vi "BracePLUS_UI_Analysis.vi"(8 "error in":errorcluster, 11 "Path":path) -> (0 "error out":errorcluster)   [LabVIEW 2018]
uses:
  <vilib>/Math Plots/3D Math Plots/3D Surface/3D Surface XCtrl/3D Surface.xctl
  subVIs/calibration/FGVs/FGV States.ctl
  <vilib>/Utility/file.llb/Read Delimited Spreadsheet (I64).vi
  <vilib>/Math Plots/3D Math Plots/3D Surface/3D Surface Datatype/Public/Plot Helper (Matrix).vi
  <vilib>/Math Plots/3D Math Plots/3D Surface/3D Surface Datatype/3D Surface Datatype.lvclass
panel:
  in  "Quit":bool
  out "Time Frame":i32(slide) scale=0.0..975.0
  in  "Tab Control":T1(tab)
  out "3D Surface":refnum<class "3D Plot Datatype.lvclass">[](xcontrol)
  out "Z Time_Integral":refnum<class "3D Plot Datatype.lvclass">[](xcontrol)
  out "Data Packet":string
  out "Time":u32=4294745741
  out "Lookup Indices":i32[](array[numeric])=[0, 4, 8, 12, 1, 5, 9, 13, 16, 20, 24, 28, 17, 21, 25, 29, 15, 11, 7, 3, 14, 10, 6, 2, 31, 27, 23, 19, 30, 26, 22, 18, 32, 36, 40, 44, 33, 37, 41, 45, 48, 52, 56, 60, 49, 53, 57, 61, 47, 43, 39, 35, 46, 42, 38, 34, 63, 59, 55, 51, 62, 58, 54, 50, 64, 68, 72, 76, 65, 69, 73, 77, 80, 84, 88, 92, 81, 85, 89, 93, 79, 75, 71, 67, 78, 74, 70, 66, 95, 91, 87, 83, 94, 90, 86, 82, 96, 100, 104, 108, 97, 101, 105, 109, 112, 116, 120, 124, 113, 117, 121, 125, 111, 107, 103, 99, 110, 106, 102, 98, 127, 123, 119, 115, 126, 122, 118, 114]
  out "EOF?":bool
  in  "Start Z_Threshold":dbl=0.1 format="%#_13g"
  in  "Calibration File":string="Magboard_Btod_new_calib"
  in  "Gains":dbl[](array[numeric])=[0.751, 0.751, 1.21]
  in  "Upper Limit":dbl=5.0 format="%#_13g"
  in  "Lower Limit":dbl format="%#_13g"
  out "Filesize (bytes)":i64
  out "No. Packets":dbl
  out "Calibrated Output":dbl[][](array[numeric])
  out "B xyz":dbl[][](array[numeric]) format="%#.0f"
  # "ESCAPES: Analysis"
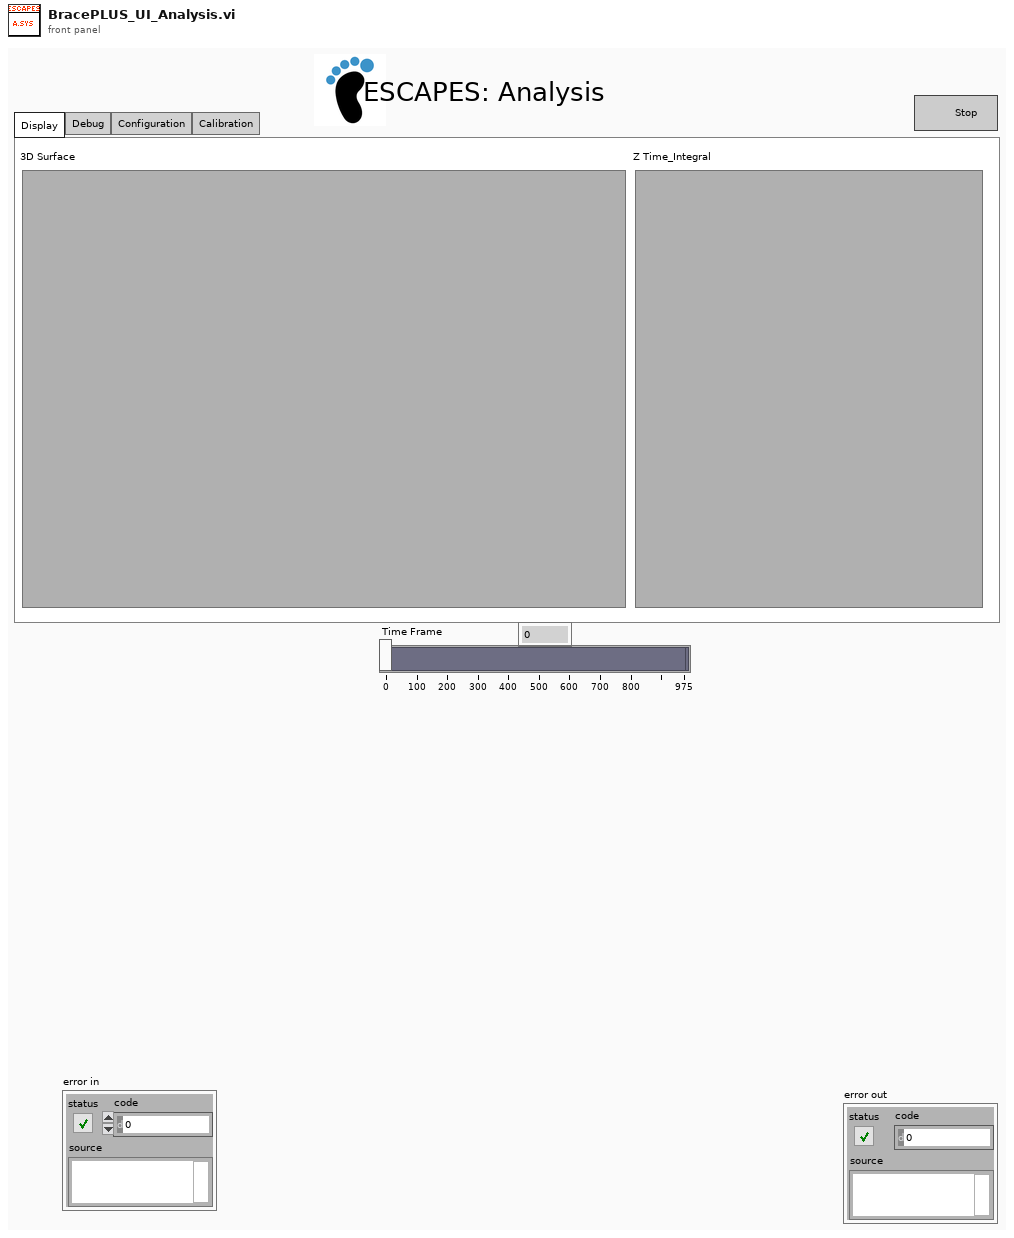
[diagram p1: front panel]
types:
  T1 = enum32{"Display", "Debug", "Configuration", "Calibration"}
  T2 = typedef "FGV States.ctl" = enum16{"Get", "Set", "Reset"}
  T3 = cluster{cluster{dbl[][], "Array":dbl[][]}, cluster{dbl[][], "Array":dbl[][]}, cluster{dbl[][], "Array":dbl[][]}, cluster{dbl[][], "Array":dbl[][]}}
  T4 = cluster{cluster{dbl[][], "Array":dbl[][]}, cluster{dbl[][], "Array":dbl[][]}, cluster{dbl[][], "Array":dbl[][]}, cluster{dbl[][], "Array":dbl[][]}}[]
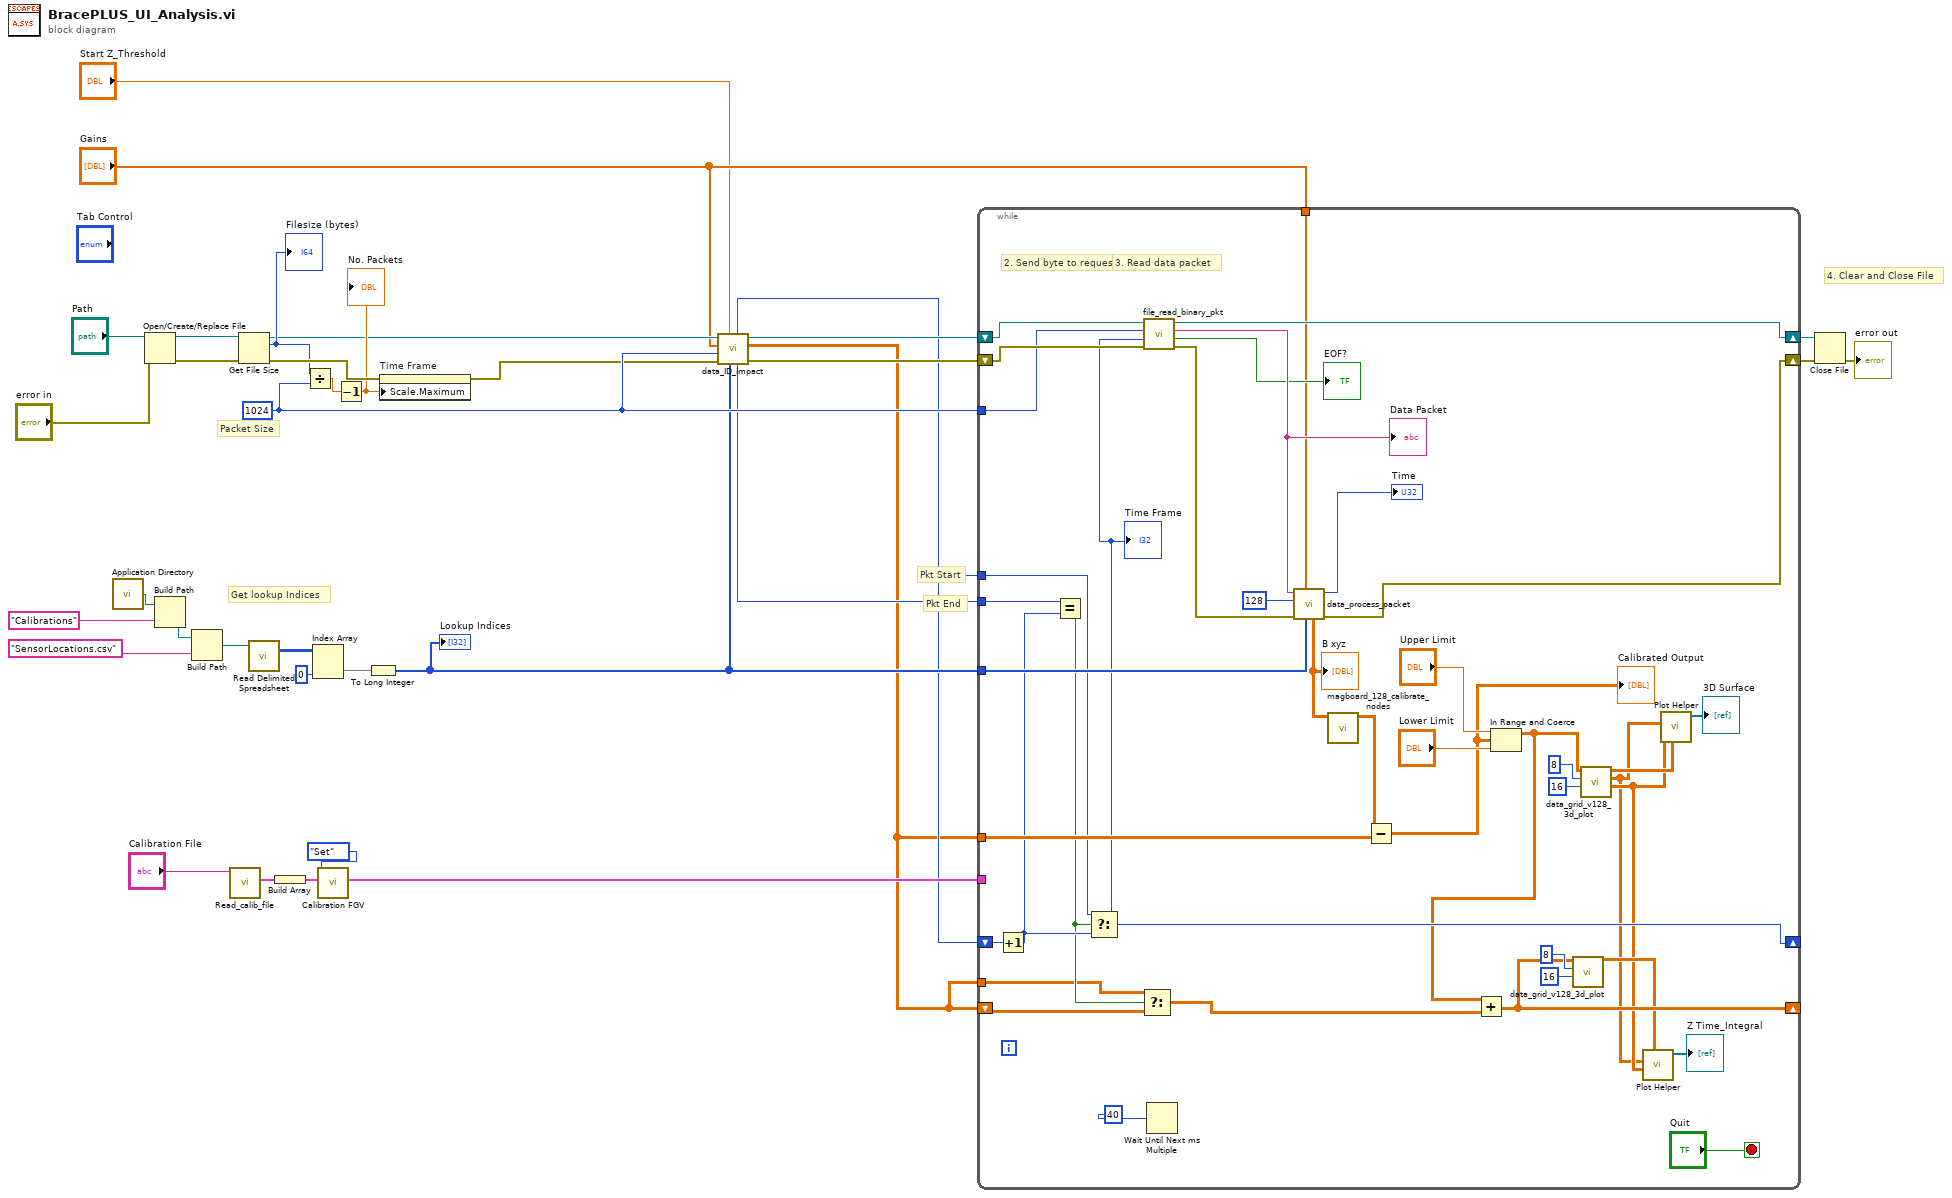
[diagram p0: block diagram]
diagram:
  w12 = 1024 ("count (1)")
  # "Pkt End"
  # "Pkt Start"
  # "Packet Size"
  # "Get lookup Indices"
  # "4. Clear and Close File"
  n1 = call <vilib>:"Application Directory.vi"() -> ("Application Directory"=w15:path)
  n2 = Open/Create/Replace File(file path (use dialog)="Path", error in="error in") -> (refnum out=w24:refnum<file>, error out=w23:errorcluster)  [unwired: 4 in, 1 out]
  n3 = Build Path(base path=w15, name or relative path="Calibrations" ("string")) -> (appended path=w17:path)
  n4 = Build Path(base path=w17, name or relative path="SensorLocations.csv" ("string")) -> (appended path=w14:path)
  n5 = call "Read_calib_file.vi"("string"="Calibration File") -> ("output cluster"=w32:T3)  [unwired: 6 in, 4 out]
  n6 = Get File Size(file=w24, error in=w23) -> (refnum out=w11:refnum<file>, size (in bytes)=w20:i64, 0:w22:errorcluster)
  "Filesize (bytes)" <- w20
  n7 = call-poly <vilib>:"Read Delimited Spreadsheet.vi"("file path (dialog if empty)"=w14) -> ("all rows"=w35:i64[][])  [unwired: 9 in, 5 out]
  n8 = Build Array(w32) -> (w31:T4)
  n9 = Divide(x=w20, y=w12) -> (x/y=w21:dbl)
  n10 = Index Array(array=w35, index (col)=0 ("disabled index (col)")) -> (element=w33:i64[])  [unwired: 1 in]
  n11 = call "Calibration FGV.vi"("Calib in"=w31, "FGV States"=FGV_States."Set") -> ("Calib in 2"=w29:T4)  [unwired: 9 in]
  n12 = Decrement(x=w21) -> (x-1=w19:dbl)
  "No. Packets" <- w19
  n13 = To Long Integer(number=w33) -> (32bit integer=w6:i32[])
  "Lookup Indices" <- w6
  n14 = property on="Time Frame" class="Slide (strict)"(error in=w22, "Scale.Maximum"=w19) -> (error out=w9:errorcluster)  [unwired: 1 in, 1 out]
  n15 = call "data_ID_impact.vi"("Sensor Lookup Indices"=w6, "Start Z_Threshold"="Start Z_Threshold", "error in (no error)"=w9, "Pkt Size"=w12, "Gains"="Gains", "Byte Stream File in"=w11) -> ("error out"=w8:errorcluster, "Sensor_Tare"=w2:dbl[][], "Byte Stream File out"=w10:refnum<file>, "N_end"=w4:i32, "N_start"=w3:i32)  [unwired: 1 in]
  n16 = while {
    shift-right: [w69] -> w26
    shift-left: w10 -> [w71]
    tunnel: w6 -> [w75]
    shift-right: [w73] -> w27
    shift-left: w8 -> [w70]
    tunnel: w29 -> [_]
    tunnel: w12 -> [w64]
    tunnel: "Gains" -> [w56]
    tunnel: w2 -> [w58]
    tunnel: w3 -> [w51]
    tunnel: w4 -> [w55]
    shift-right: [w50] -> _
    shift-left: w3 -> [w53]
    shift-right: [w45] -> _
    shift-left: w2 -> [w39]
    tunnel: w2 -> [w40]
    stop <- "Quit" stop-if-true
    # "3. Read data packet"
    # "2. Send byte to request reading"
    n17 = Increment(x=w53) -> (x+1=w52:i32)
    n18 = Equal?(x=w55, y=w52) -> (x = y?=w41:bool)
    n19 = Select(t=w51, s=w41, f=w52) -> (s? t:f=w50:i32)
    "Time Frame" <- w50
    n20 = Select(t=w40, s=w41, f=w39) -> (s? t:f=w38:dbl[][])
    n21 = call "file_read_binary_pkt.vi"("error in (no error)"=w70, "Packet No."=w50, "Pkt Size(bytes)"=w64, "Byte Stream File in"=w71) -> ("error out"=w68:errorcluster, "EOF?"=→"EOF?":bool, "Packet"=w65:string, "Byte Stream File out"=w69:refnum<file>)  [unwired: 4 in]
    "Data Packet" <- w65
    n22 = Wait Until Next ms Multiple(millisecond multiple=u32 40 ("Playback dT")) -> ()  [unwired: 1 out]
    n23 = call "data_process_packet.vi"("Sensor Lookup Indices"=w75, "Gains"=w56, "error in (no error)"=w68, "No. Sensors"=128 ("No. Nodes"), "Binary Input Data"=w65) -> ("error out"=w73:errorcluster, "Time"=→"Time":u32, "Sensors (uT)"=w72:dbl[][])  [unwired: 2 in, 2 out]
    "B xyz" <- w72
    n24 = call "magboard_128_calibrate_nodes.vi"("Sensor Input (mT)"=w72) -> ("Sensor Output - Position (mm)"=w60:dbl[][])  [unwired: 10 in]
    n25 = Subtract(x=w60, y=w58) -> (x-y=w48:dbl[][])
    "Calibrated Output" <- w48
    n26 = In Range and Coerce(upper limit="Upper Limit", x=w48, lower limit="Lower Limit") -> (coerced(x)=w36:dbl[][])  [unwired: 1 out]
    n27 = Add(x=w36, y=w38) -> (x+y=w45:dbl[][])
    n28 = call "data_grid_v128_3d_plot.vi"("No. Rows"=16 ("Row Length"), "No. Columns"=8, "Sensor Data"=w45) -> ("Z (GRID)"=w44:dbl[][])  [unwired: 6 in, 2 out]
    n29 = call "data_grid_v128_3d_plot.vi"("No. Rows"=16 ("Row Length"), "No. Columns"=8, "Sensor Data"=w36) -> ("Y (GRID)"=w43:dbl[][], "X (GRID)"=w42:dbl[][], "Z (GRID)"=w61:dbl[][])  [unwired: 6 in]
    n30 = call-poly <vilib>:"Plot Helper.vi"("z matrix"=w44, "y matrix"=w43, "x matrix"=w42) -> ("3D Plot lvclass Array out"=→"Z Time_Integral":refnum<class "3D Plot Datatype.lvclass">[])  [unwired: 3 in, 5 out]
    n31 = call-poly <vilib>:"Plot Helper.vi"("z matrix"=w61, "y matrix"=w43, "x matrix"=w42) -> ("3D Plot lvclass Array out"=→"3D Surface":refnum<class "3D Plot Datatype.lvclass">[])  [unwired: 3 in, 5 out]
  }
  n32 = Close File(refnum=w26, error in=w27) -> (error out=→"error out":errorcluster)  [unwired: 1 out]
